vi "Flatten UTC.vi"(11 "Local Time in":timestamp) -> (3 "Sec Hdr TLM":T1)   [LabVIEW 2018, in "TCPServer.lvlib"]
uses:
  TCPServer.lvlib
  TypeDefs/Sec Hdr TLM.ctl
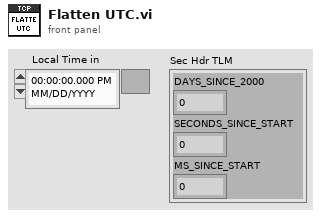
[diagram p1: front panel]
types:
  T1 = typedef "TCPServer.lvlib/Sec Hdr TLM.ctl" = cluster{"DAYS_SINCE_2000":u16, "SECONDS_SINCE_START":u32, "MS_SINCE_START":u16}
  T2 = typedef "LVDateTimeRec.ctl" = cluster{"fractional second":dbl, "second":i32, "minute":i32, "hour":i32, "day of month":i32, "month":i32, "year":i32, "day of week":i32, "day of year":i32, "DST":i32}
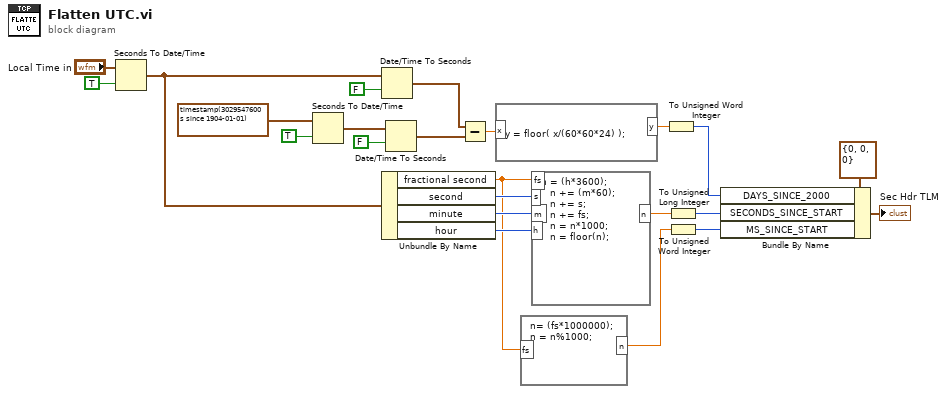
[diagram p0: block diagram]
diagram:
  n1 = Seconds To Date/Time(time stamp (now)="Local Time in", to UTC (F)=TRUE) -> (date time rec=w13:T2)
  n2 = Seconds To Date/Time(time stamp (now)=timestamp(3029547600 s since 1904-01-01), to UTC (F)=TRUE) -> (date time rec=w20:T2)
  n3 = Date/Time To Seconds(1:FALSE, 2:w13) -> (0:w14:timestamp)
  n4 = Unbundle By Name(w13) -> ("fractional second"=w7:dbl, "second"=w10:i32, "minute"=w11:i32, "hour"=w12:i32)
  n5 = Date/Time To Seconds(1:FALSE, 2:w20) -> (0:w17:timestamp)
  n6 = Subtract(x=w14, y=w17) -> (x-y=w4:dbl)
  n7 = formula code="y = floor( x/(60*60*24) );"("x"=w4) -> ("y"=w16:dbl)
  n8 = formula code="n= (fs*1000000);\nn = n%1000;"("fs"=w7) -> ("n"=w6:dbl)
  n9 = formula code="n = (h*3600);\n   n += (m*60);\n   n += s;\n   n += fs;\n   n = n*1000;\n   n = floor(n);"("m"=w11, "h"=w12, "s"=w10, "fs"=w7) -> ("n"=w9:dbl)
  n10 = To Unsigned Word Integer(number=w16) -> (unsigned 16bit integer=w15:u16)
  n11 = To Unsigned Long Integer(number=w9) -> (unsigned 32bit integer=w8:u32)
  n12 = To Unsigned Word Integer(number=w6) -> (unsigned 16bit integer=w5:u16)
  n13 = Bundle By Name(cluster=T1 {"DAYS_SINCE_2000"=0, "SECONDS_SINCE_START"=0, "MS_SINCE_START"=0} ("SecHdrTLM"), "DAYS_SINCE_2000"=w15, "SECONDS_SINCE_START"=w8, "MS_SINCE_START"=w5) -> (→"Sec Hdr TLM":T1)
